vi "Control, Set Next Y.vi"(5 "margin (16)":i32=16, 6 "error in":errorcluster, 8 "Ctl ref2":refnum<vi>, 9 "Ctl ref1":refnum<vi>) -> (0 "error out":errorcluster, 2 "Ctl ref dup2":refnum<vi>, 3 "Ctl ref dup1":refnum<vi>)   [LabVIEW 2010]
doc: "This function sets the vertical position of a GUI control relative to a GUI control reference."
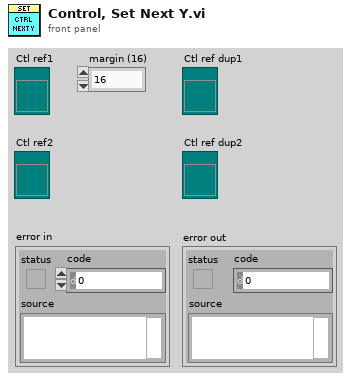
[diagram p1: front panel]
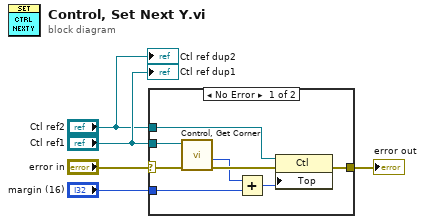
[diagram p0: block diagram]
diagram:
  n1 = case shown="No Error" "error in" {
    selector: "error in" -> [w9 w14]
    tunnel: [w12 w14] -> w5
    tunnel: "Ctl ref1" -> [w6 _]
    tunnel: "margin (16)" -> [w11 _]
    tunnel: "Ctl ref2" -> [w10 _]
    frame No Error {
      n2 = call "Control, Get Corner.vi"("error in"=w9, "Ctl ref"=w6) -> ("error out"=w8:errorcluster, "bottom"=w7:i32)  [unwired: 4 in, 2 out]
      n3 = Add(x=w7, y=w11) -> (x+y=w13:i32)
      n4 = property class="Ctl"(reference=w10, error in=w8, "Top"=w13) -> (error out=w12:errorcluster)  [unwired: 1 out]
    }
    frame Error {
    }
  }
  "error out" <- w5
  "Ctl ref dup1" <- "Ctl ref1"
  "Ctl ref dup2" <- "Ctl ref2"
